vi "_Release JKISMQ.vi"(8 "Error in":errorcluster caption="Error in (no error)", 11 "JKISMQ":T1) -> (0 "Error out":errorcluster)   [LabVIEW 2014, in "JKI-State-Machine-Plus.lvlib"]
uses:
  JKI-State-Machine-Plus.lvlib
  _JKISMQ.ctl
  Typedef/_Cross JKI StateMachine State Data.ctl
  Typedef/_JKISM_MSG_TYPE.ctl
  Typedef/_Cross JKI StateMachine State Response.ctl
  FGV-BroadcastRegistry/Oper-BroadcastRegistry.ctl
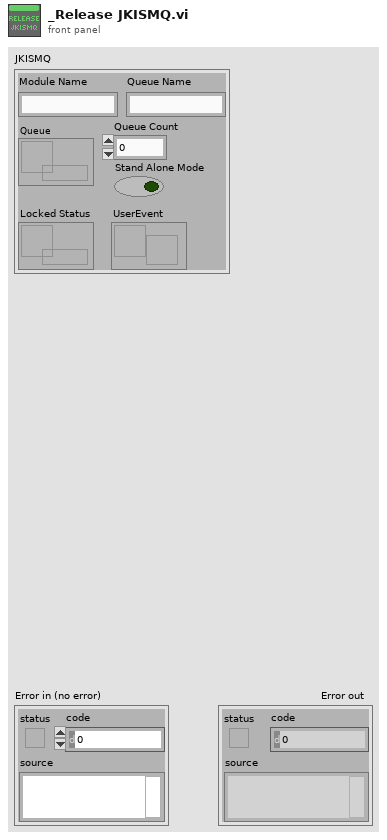
[diagram p1: front panel]
types:
  T1 = typedef "JKI-State-Machine-Plus.lvlib/_JKISMQ.ctl" = cluster{"Module Name":string, "Queue":refnum<queue>, "Locked Status":refnum<data-value>, "Stand Alone Mode":bool, "UserEvent":refnum<user-event>, "Queue Name":string, "Queue Count":i32}
  T2 = typedef "JKI-State-Machine-Plus.lvlib/Oper-BroadcastRegistry.ctl" = enum16{"Delete Source Module", "Delete Dest Module", "Remove Module", "Register", "Unregister", "Check"}
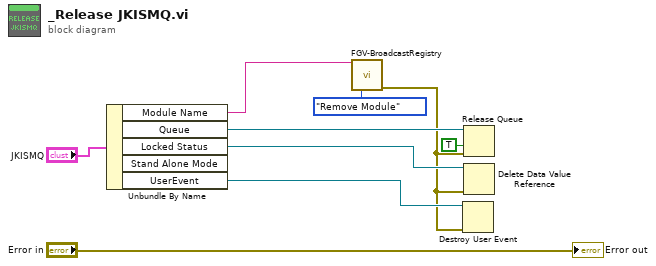
[diagram p0: block diagram]
diagram:
  n1 = Unbundle By Name("JKISMQ") -> ("Module Name"=w2:string, "Queue"=w7:refnum<queue>, "Locked Status"=w5:refnum<data-value>, "UserEvent"=w4:refnum<user-event>)  [unwired: 1 out]
  n2 = call "FGV-BroadcastRegistry.vi"("Source"=w2, "Operation"=Oper-BroadcastRegistry."Remove Module") -> ("Error out"=w1:errorcluster)  [unwired: 11 in, 2 out]
  n3 = Destroy User Event(user event=w4, error in=w1) -> ()  [unwired: 1 out]
  n4 = Release Queue(queue=w7, force destroy? (F)=TRUE, error in (no error)=w1) -> ()  [unwired: 3 out]
  n5 = Delete Data Value Reference(data value reference=w5, error in=w1) -> ()  [unwired: 2 out]
  "Error out" <- "Error in"
